vi "TestRaspiComm.vi"() -> ()   [LabVIEW 2019]
uses:
  <vilib>/Instr/_visa.llb/VISA Configure Serial Port (Serial Instr).vi
panel:
  out "Response":string[](array[string])
  in  "stop":bool
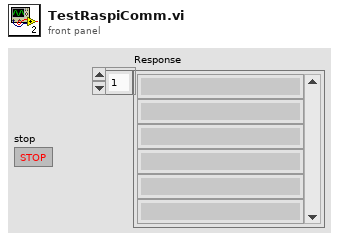
[diagram p1: front panel]
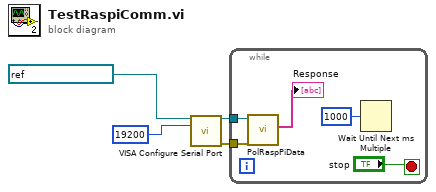
[diagram p0: block diagram]
diagram:
  n1 = call-poly "VISA Configure Serial Port"("VISA resource name"=refnum<visa-resource-name> "ASRL12::INSTR" ("VISA Sesssion In"), "baud rate (9600)"=u32 19200) -> ("VISA resource name out"=w3:refnum<visa-resource-name>, "error out"=w1:errorcluster)  [unwired: 12 in]
  n2 = while {
    tunnel: w3 -> [w9]
    tunnel: w1 -> [w8]
    stop <- "stop" stop-if-true
    n3 = call "PolRaspPiData.vi"("error in (no error)"=w8, "VISA Sesssion In"=w9) -> ("output array"=→"Response":string[])  [unwired: 7 in, 2 out]
    n4 = Wait Until Next ms Multiple(millisecond multiple=u32 1000) -> ()  [unwired: 1 out]
  }
